vi "numeric.vi"() -> ()   [LabVIEW 2019]
panel:
  out "absolute":dbl
  out "?":dbl
  out "reciprocal":dbl
  out "negate":dbl
  out "square":dbl
  out "sq root":dbl
  out "scale by  power":dbl
  out "decremen":dbl
  out "increment":dbl
  out "divide":dbl
  out "multi":dbl
  out "sub":dbl
  out "add":dbl
  in  "y":dbl
  in  "x":dbl
  # "round to nearest"
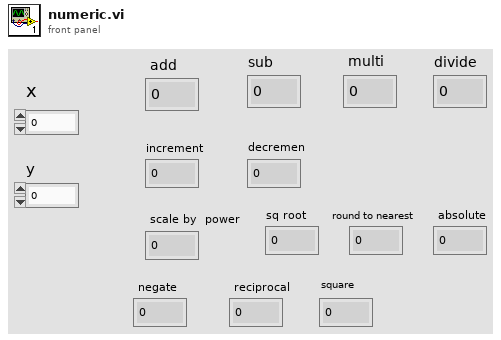
[diagram p1: front panel]
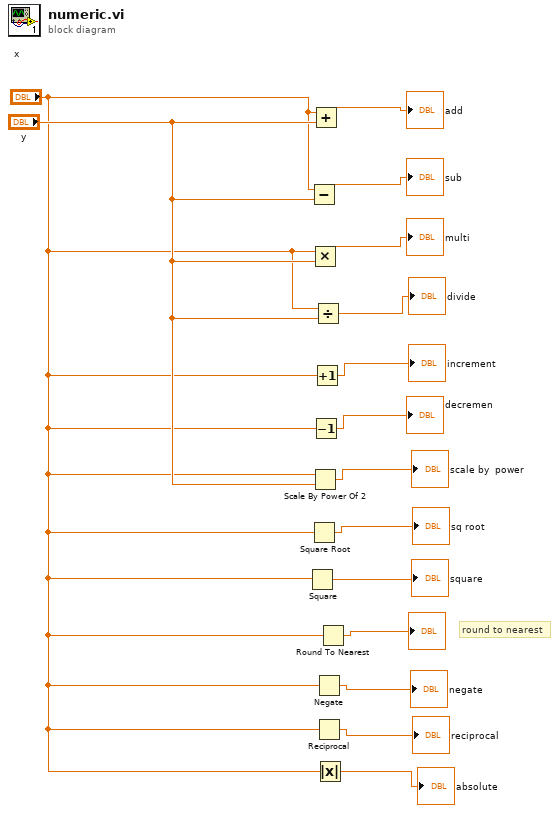
[diagram p0: block diagram]
diagram:
  # "round to nearest"
  n1 = Square(x="x") -> (x^2=→"square":dbl)
  n2 = Subtract(x="x", y="y") -> (x-y=→"sub":dbl)
  n3 = Square Root(x="x") -> (sqrt(x)=→"sq root":dbl)
  n4 = Multiply(x="x", y="y") -> (x*y=→"multi":dbl)
  n5 = Scale By Power Of 2(n="x", x="y") -> (x*2^n=→"scale by  power":dbl)
  n6 = Add(x="x", y="y") -> (x+y=→"add":dbl)
  n7 = Decrement(x="x") -> (x-1=→"decremen":dbl)
  n8 = Increment(x="x") -> (x+1=→"increment":dbl)
  n9 = Divide(x="x", y="y") -> (x/y=→"divide":dbl)
  n10 = Negate(x="x") -> (-x=→"negate":dbl)
  n11 = Reciprocal(x="x") -> (1/x=→"reciprocal":dbl)
  n12 = Absolute Value(x="x") -> (abs(x)=→"absolute":dbl)
  n13 = Round To Nearest(number="x") -> (nearest integer value=→"?":dbl)
